vi "Plugin Page GUID.vi"() -> (3 "Plugin GUID":string="e36400aa-5528-4ac8-8885-6b99ede07395")   [LabVIEW 2017, in "DSF Shared.lvlib"]
uses:
  DSF Shared.lvlib
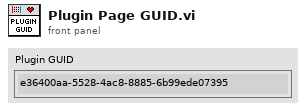
[diagram p1: front panel]
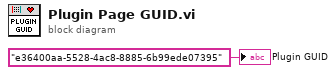
[diagram p0: block diagram]
diagram:
  "Plugin GUID" <- "e36400aa-5528-4ac8-8885-6b99ede07395" ("Data Sharing Framework")
